vi "POST MesaurementsMappingTable.vi"(8 "error in":errorcluster, 11 "GTron in":path) -> (0 "error out":errorcluster, 3 "DB is Empty?":bool)   [LabVIEW 2019, in "DataLogger.lvclass"]
doc: "POST Measurement Mapping Table"
uses:
  DataLogger.lvclass
  <vilib>/httpClient/LabVIEWHTTPClient.lvlib
  <vilib>/drjdpowell/SQLite Library/SQL Statement/SQL Statement.lvclass
  <vilib>/drjdpowell/SQLite Library/SQL Connection/Open (path).vi
  <vilib>/drjdpowell/SQLite Library/SQL Connection/Execute SQL (Single Integer).vi
  <vilib>/httpClient/POSTBuffer.vi
  <vilib>/drjdpowell/SQLite Library/SQL Connection/Connection.lvclass
  <vilib>/drjdpowell/SQLite Library/SQL Connection/Execute SQL (No results).vi
panel:
  in  "Measurement Keys in":string[](array[string])=["PartName", "MeasurementName", "LSL", "USL", "LCL", "UCL", "InspectionMcId", "Status", "NominalValue"]
  in  "Server info Cluster for Measurement in":T1={"JSON Buffer"="authtoken=47244d7c61d7e6141acdddeabbf622d1&scope=creatorapi&zc_ownername=zentron3&XMLString=", "Server information start tag"="<ZohoCreator> <applicationlist> <application name='iiot-gtron'><formlist>  <form name='SimulatedPartsMeasurementsMapping'>", "Record start/end"="add", "Key name"="field name", "Value name"="value", "Server information end tag"="\"</form></formlist></application></applicationlist></ZohoCreator>"}
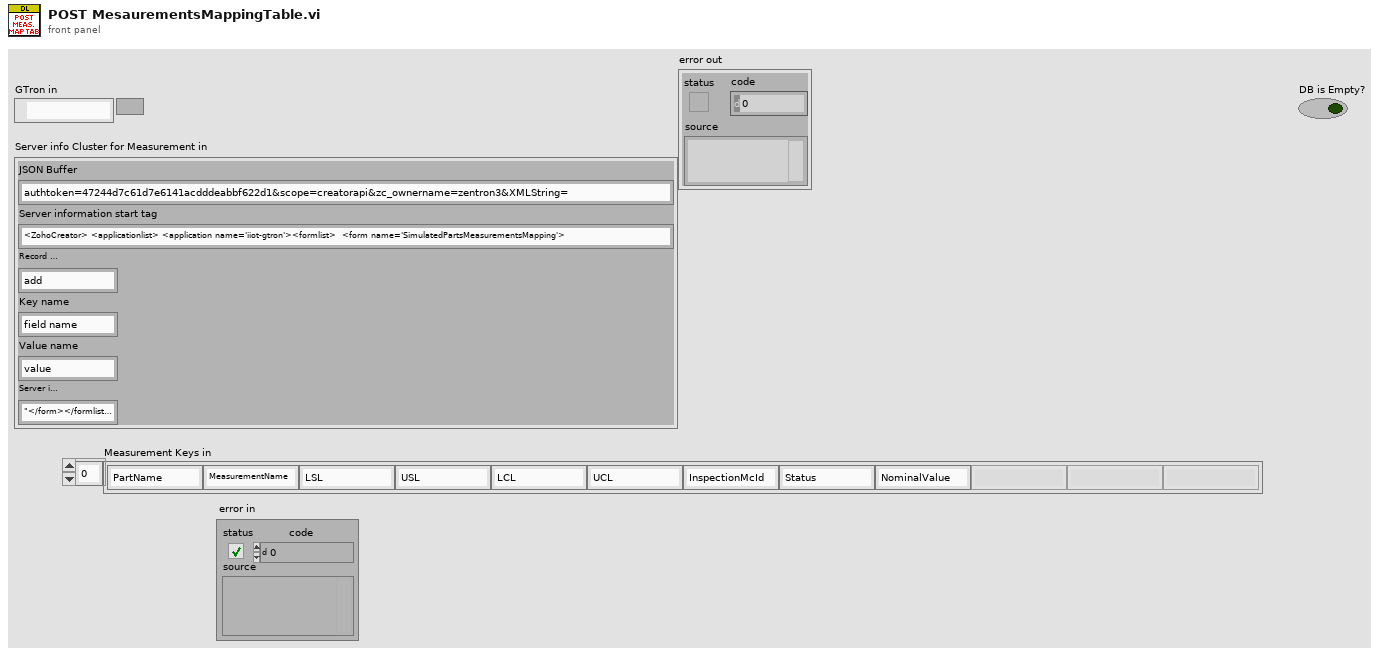
[diagram p1: front panel]
types:
  T1 = cluster{"JSON Buffer":string, "Server information start tag":string, "Record start/end":string, "Key name":string, "Value name":string, "Server information end tag":string}
  T2 = typedef "LabVIEWHTTPClient.lvlib/ClientHandle.ctl" = refnum<k1>
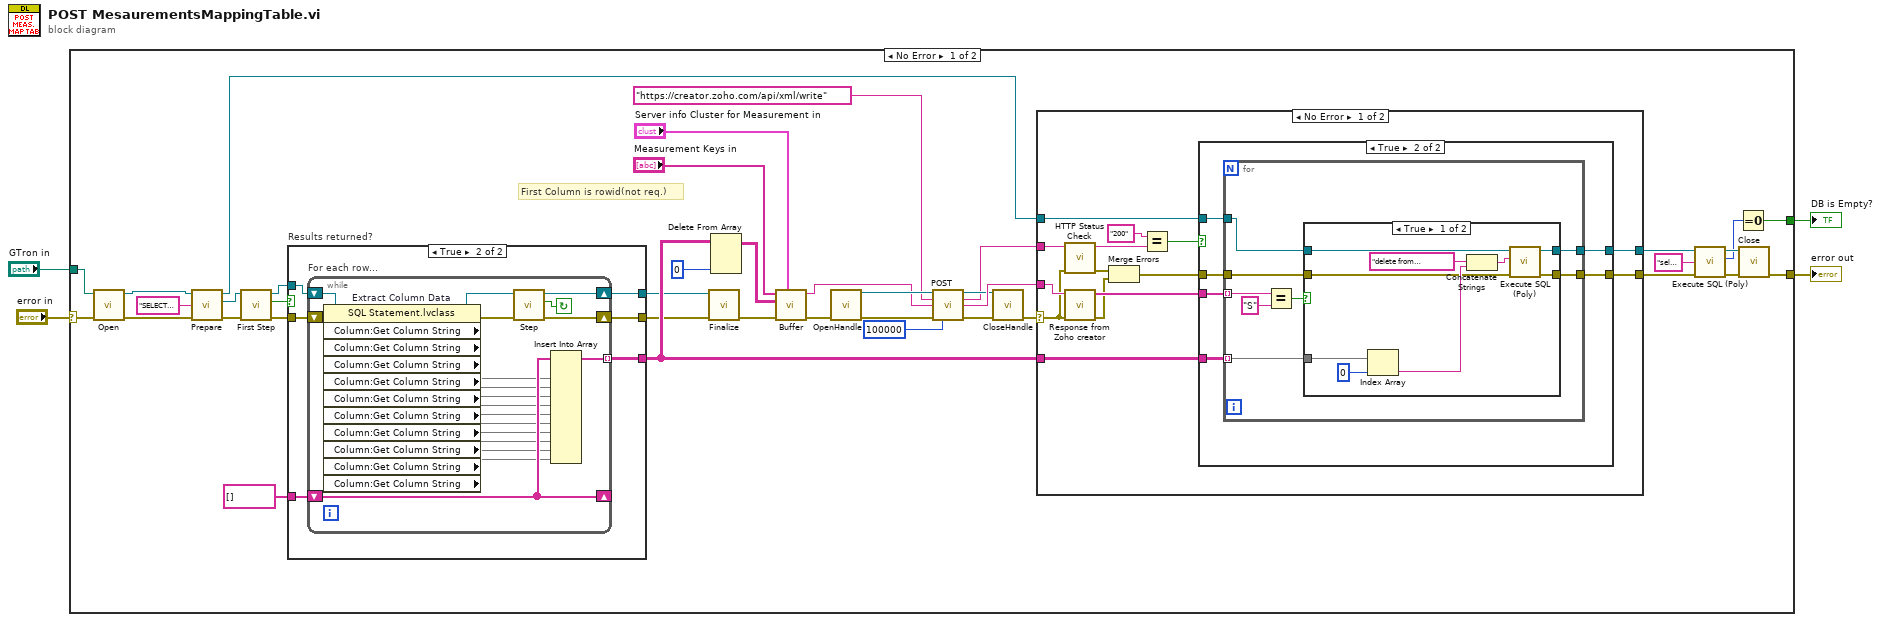
[diagram p0: block diagram]
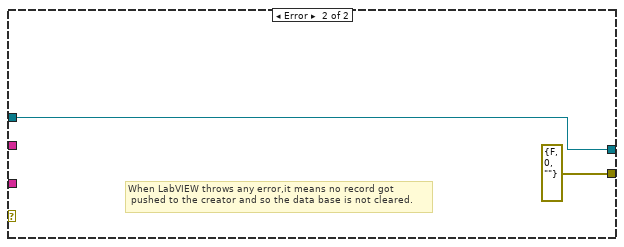
[diagram p5: hidden frame]
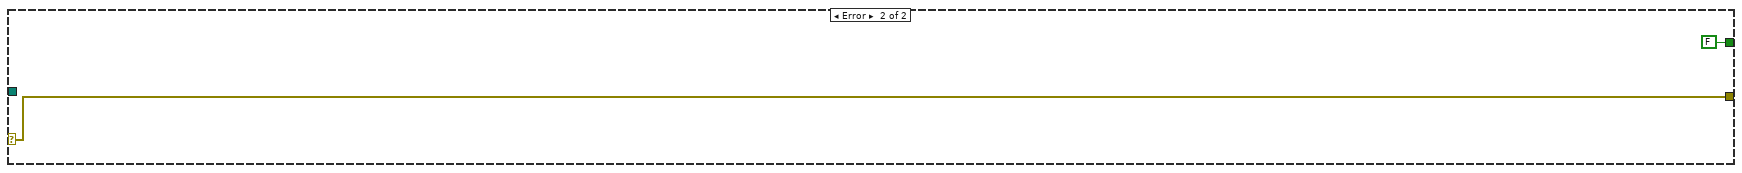
[diagram p6: hidden frame]
diagram:
  n1 = case shown="No Error" "error in" {
    selector: "error in" -> [w7 w115]
    tunnel: "GTron in" -> [w18 _]
    tunnel: [w8 w115] -> w3
    tunnel: [w5 FALSE] -> w1
    frame No Error {
      # "First Column is rowid(not req.)"
      n2 = call-poly <vilib>:"Open.vi"("error in (no error)"=w7, "db file"=w18) -> ("error out"=w38:errorcluster, "SQLite Connection"=w37:refnum<class "Connection.lvclass">)  [unwired: 8 in]
      n3 = call <vilib>:"Prepare.vi"("error in (no error)"=w38, "SQL"="SELECT rowid,PartName,MeasurementName,LSL,USL,LCL,UCL,InspectionMcId,Status,NominalValue FROM PartsMeasurementMapping" ("SELECT  statement"), "SQLite Connection in"=w37) -> ("error out"=w16:errorcluster, "SQL Statement"=w12:refnum<class "SQL Statement.lvclass">, "SQLite Connection"=w23:refnum<class "Connection.lvclass">)  [unwired: 4 in, 2 out]
      n4 = call <vilib>:"First Step.vi"("error in (no error)"=w16, "SQL Statement in"=w12) -> ("error out"=w14:errorcluster, "Row returned"=w15:bool, "SQL Statement"=w13:refnum<class "SQL Statement.lvclass">)  [unwired: 7 in]
      n5 = case "Results returned?" shown="True" w15 {
        tunnel: [w45 w51] -> w11
        tunnel: [w44 w50] -> w10
        tunnel: w13 -> [w45 w49]
        tunnel: w14 -> [w44 w48]
        tunnel: string[] [] -> [_ w47]
        tunnel: [_ w46] -> w22
        frame False {
        }
        frame True {
          n6 = while "For each row..." {
            shift-right: [w69] -> w51
            shift-left: w49 -> [w66]
            shift-right: [w67] -> w50
            shift-left: w48 -> [w65]
            shift-right: [w64] -> _
            shift-left: w47 -> [w64]
            tunnel: [w57] -> w46 mode=indexing
            stop <- w55 continue-if-true
            n7 = property on="Extract Column Data" class="SQL Statement.lvclass"(reference=w66, error in=w65) -> (reference out=w70:refnum<class "SQL Statement.lvclass">, error out=w68:errorcluster, "Column:Get Column String"=w56, "Column:Get Column String"=w63, "Column:Get Column String"=w62, "Column:Get Column String"=w61, "Column:Get Column String"=w60, "Column:Get Column String"=w59, "Column:Get Column String"=w58, "Column:Get Column String"=w54, "Column:Get Column String"=w53, "Column:Get Column String"=w52)
            n8 = call <vilib>:"Step.vi"("error in (no error)"=w68, "SQL Statement in"=w70) -> ("error out"=w67:errorcluster, "Row returned"=w55:bool, "SQL Statement"=w69:refnum<class "SQL Statement.lvclass">)  [unwired: 7 in]
            n9 = Insert Into Array(array=w64, new element #1=w56, new element #2=w63, new element #3=w62, new element #4=w61, new element #5=w60, new element #6=w59, new element #7=w58, new element #8=w54, new element #9=w53, new element #10=w52) -> (w57:string[])  [unwired: 1 in]
          }
        }
      }
      n10 = call <vilib>:"Finalize.vi"("error in (no error)"=w10, "SQL Statement in"=w11) -> ("error out"=w39:errorcluster)  [unwired: 9 in]
      n11 = Delete From Array(array=w22, index (col)=0 ("disabled index (col)")) -> (array with subset deleted=w35:string[][])  [unwired: 2 in, 1 out]
      n12 = call "Buffer.vi"("Cluster"="Server info Cluster for Measurement in", "error in"=w39, "Values"=w35, "Keys"="Measurement Keys in") -> ("Error out"=w40:errorcluster, "Buffer"=w30:string)  [unwired: 6 in]
      n13 = call <vilib>:"OpenHandle.vi"("error in (no error)"=w40) -> ("client handle out"=w32:T2, "error out"=w27:errorcluster)  [unwired: 13 in]
      n14 = call-poly <vilib>:"POST.vi"("client handle"=w32, "url"="https://creator.zoho.com/api/xml/write", "buffer"=w30, "error in (no error)"=w27, "timeout (10000)"=100000) -> ("client handle out"=w31:T2, "headers"=w24:string, "body"=w41:string, "error out"=w26:errorcluster)  [unwired: 7 in]
      n15 = call <vilib>:"CloseHandle.vi"("client handle"=w31, "error in (no error)"=w26) -> ("error out"=w25:errorcluster)  [unwired: 13 in]
      n16 = case shown="No Error" w25 {
        selector: w25 -> [w75 _]
        tunnel: w24 -> [w84 _]
        tunnel: w41 -> [w77 _]
        tunnel: w23 -> [w80 w113]
        tunnel: w22 -> [w79 _]
        tunnel: [w78 w113] -> w20
        tunnel: [w71 errorcluster {"status"=FALSE, "code"=0, "source"=""} ("error out")] -> w42
        frame No Error {
          n17 = call "HTTP Status Check.vi"("error in (no error)"=w75, "String"=w84) -> ("error out"=w74:errorcluster, "HTTP Status Code"=w83:string)  [unwired: 7 in]
          n18 = call "Response from Zoho creator.vi"("error in"=w75, "body"=w77) -> ("error out"=w73:errorcluster, "decimated array"=w76:string[])  [unwired: 8 in]
          n19 = Merge Errors(w74, w73) -> (w72:errorcluster)
          n20 = Equal?(x="200" ("y"), y=w83) -> (x = y?=w81:bool)
          n21 = case shown="True" w81 {
            tunnel: w76 -> [_ w91]
            tunnel: w80 -> [w86 w92]
            tunnel: w79 -> [_ w90]
            tunnel: [w86 w89] -> w78
            tunnel: w72 -> [w85 w88]
            tunnel: [w85 w87] -> w71
            frame False {
              # "When HTTP Status is anything except 200,it means no record\ngot pushed to the creator and so the database is not cleared"
            }
            frame True {
              n22 = for {
                tunnel: w92 -> [w100]
                tunnel: w90 -> [w96] mode=indexing
                tunnel: w91 -> [w99] mode=indexing
                tunnel: [w95] -> w89
                tunnel: w88 -> [w94]
                tunnel: [w93] -> w87
                n23 = Equal?(x=w99, y="S") -> (x = y?=w97:bool)
                n24 = case shown="True" w97 {
                  tunnel: w100 -> [w109 w111]
                  tunnel: w96 -> [w108 _]
                  tunnel: [w103 w111] -> w95
                  tunnel: w94 -> [w102 w110]
                  tunnel: [w101 w110] -> w93
                  frame True {
                    n25 = Index Array(array=w108, index=0) -> (element=w106:string)
                    n26 = Concatenate Strings("delete from PartsMeasurementMapping where rowid = " ("SQL"), w106) -> (w104:string)
                    n27 = call-poly <vilib>:"Execute SQL (Poly).vi"("error in (no error)"=w102, "SQL"=w104, "SQLite Connection in"=w109) -> ("error out"=w101:errorcluster, "SQLite Connection"=w103:refnum<class "Connection.lvclass">)  [unwired: 7 in]
                  }
                  frame False {
                  }
                }
              }
            }
          }
        }
        frame Error {
          # "When LabVIEW throws any error,it means no record got\n pushed to the creator and so the data base is not cleared."
        }
      }
      n28 = call-poly <vilib>:"Execute SQL (Poly).vi"("error in (no error)"=w42, "SQL"="select count(*) from PartsMeasurementMapping ", "SQLite Connection in"=w20) -> ("error out"=w43:errorcluster, "Result"=w6:i64, "SQLite Connection"=w19:refnum<class "Connection.lvclass">)  [unwired: 6 in]
      n29 = Equal To 0?(x=w6) -> (x = 0?=w5:bool)
      n30 = call-dynamic "Close.vi"("error in (no error)"=w43, "SQLite Connection in"=w19) -> ("error out"=w8:errorcluster)  [unwired: 9 in]
    }
    frame Error {
    }
  }
  "error out" <- w3
  "DB is Empty?" <- w1
